vi "Test Call Sandbox.vi"   [LabVIEW 2024]
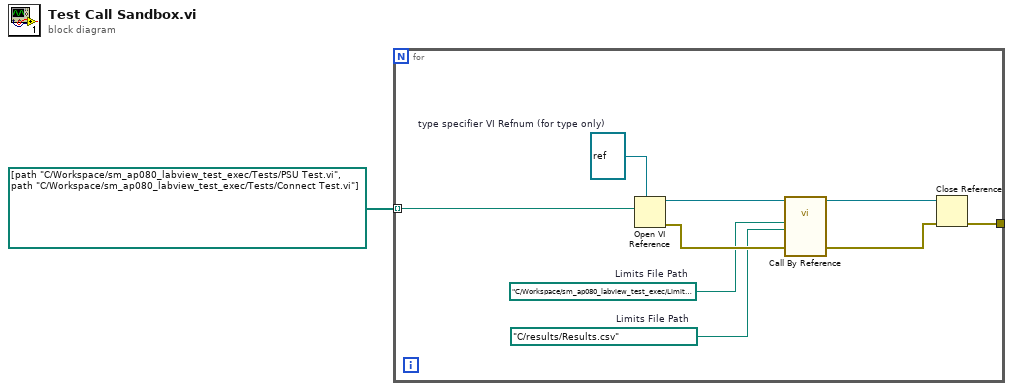
[diagram p0: block diagram]
diagram:
  n1 = for {
    tunnel: path[] [path "C:/Workspace/sm_ap080_labview_test_exec/Tests/PSU Test.vi", path "C:/Workspace/sm_ap080_labview_test_exec/Tests/Connect Test.vi"] -> [w10] mode=indexing
    tunnel: [w9] -> _
    w2 = path "C:/results/Results.csv"  # Limits File Path
    w3 = path "C:/Workspace/sm_ap080_labview_test_exec/Limits/Test Sequence V1 Limits.csv"  # Limits File Path
    w8 = refnum<vi> refnum  # type specifier VI Refnum (for type only)
    n2 = Open VI Reference(type specifier VI Refnum (for type only)=w8, vi path=w10) -> (vi reference=w7:refnum<vi>, error out=w6:errorcluster)  [unwired: 4 in]
    n3 = call-by-ref "?"(reference=w7, "Limits File Path"=w3, "Results File Path"=w2, "error in"=w6) -> (reference out=w4:refnum<vi>, "error out"=w5:errorcluster)  [unwired: 13 in, 1 out]
    n4 = Close Reference(reference=w4, error in (no error)=w5) -> (error out=w9:errorcluster)
  }
